vi "State_Launch_FPGA.vi"(8 "error in (no error)":T1, 9 "FPGA":refnum, 10 "Resource Name":string, 11 "launcher in":class) -> (0 "error out":T1, 2 "Debug Message":string, 3 "launcher out":class)   [LabVIEW 2021, in "launcher.lvclass"]
uses:
  launcher.lvclass
  <vilib>/FPGAPlugInAG/cRIO-9045/niLvFpga_Open_cRIO-9045.vi
  <vilib>/rvi/interface/common/dynamic/niFpgaDynamicAddResources.vi
  <userlib>/S2 Labs/Module Framework/Modules/Base/Module.lvclass
  <vilib>/rvi/interface/nirviOpenFPGA/nirviOpenFPGA.xnode
  cRIO_Argus-Hybrid-Vessel/FPGA Bitfiles/FPGA_9045.lvbitx
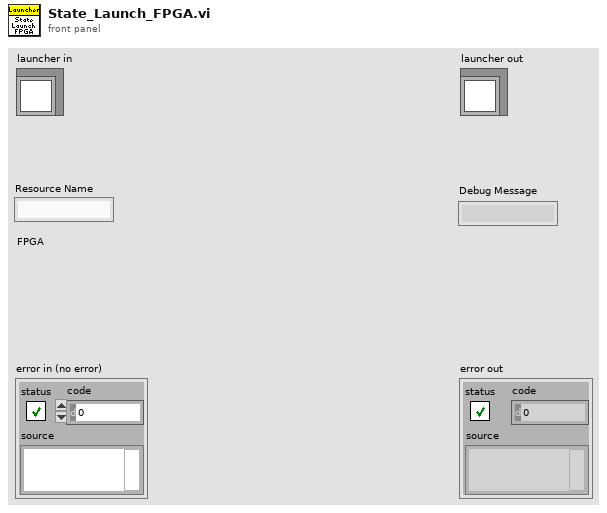
[diagram p1: front panel]
types:
  T1 = cluster{"source":string, "code":numeric, "status":boolean}
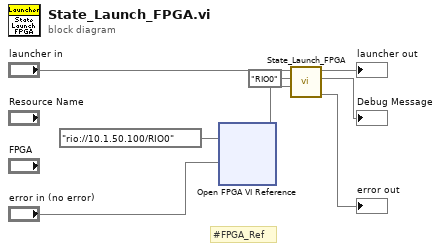
[diagram p0: block diagram]
diagram:
  # "#FPGA_Ref"
  n1 = xnode ("Open FPGA VI Reference")("error in (no error)", "rio://10.1.50.100/RIO0" ("resource name")) -> (w2)  [unwired: 1 out]
  n2 = call-parent "State_Launch_FPGA.vi"(9:w2, 10:"RIO0" ("Resource Name"), 11:"launcher in") -> (0:→"error out", 2:→"Debug Message", 3:→"launcher out")  [unwired: 6 in]
